vi "GetParam.vi"(8 "error in (no error)":errorcluster caption="entrée d'erreur (pas d'erreur)", 11 "Homogeneity_C_V_M.lvclass":refnum<class "Homogeneity_C_V_M.lvclass">) -> (0 "error out":errorcluster caption="sortie d'erreur", 2 "homogeneity_completeness_v_measure":cluster{"beta":dbl, "Returns":string}={"beta"=1.0, "Returns"="homogeneity"}, 3 "Homogeneity_C_V_M.lvclass":refnum<class "Homogeneity_C_V_M.lvclass">)   [LabVIEW 2020, in "Homogeneity_C_V_M.lvclass"]
doc: "Get parameters"
uses:
  Homogeneity_C_V_M.lvclass
  Homogeneity_C_V_M.lvclass/Homogeneity_C_V_M.ctl
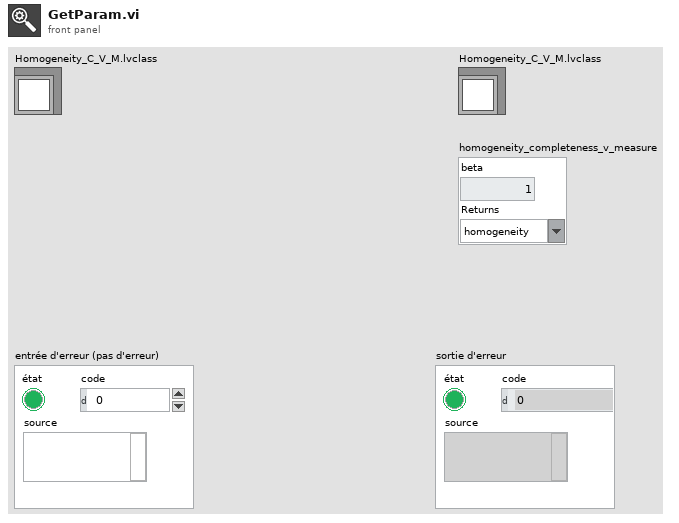
[diagram p1: front panel]
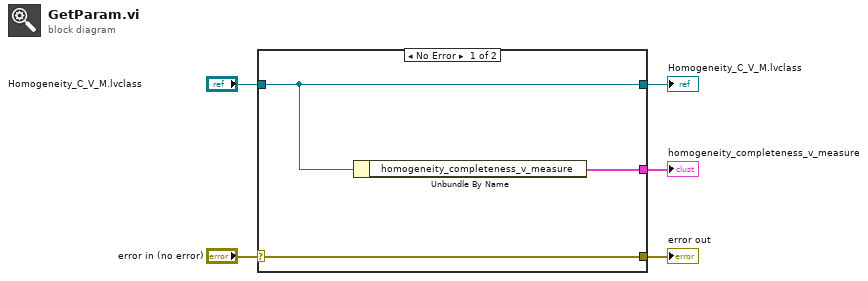
[diagram p0: block diagram]
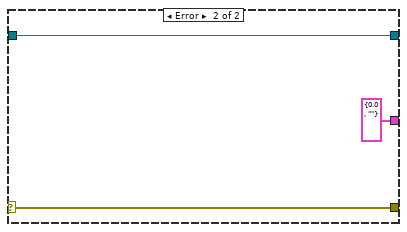
[diagram p2: hidden frame]
diagram:
  n1 = case shown="No Error" "error in (no error)" {
    selector: "error in (no error)" -> [w8 w10]
    tunnel: [w8 w10] -> w4
    tunnel: [w7 w11] -> w2
    tunnel: "Homogeneity_C_V_M.lvclass" -> [w7 w11]
    tunnel: [w6 cluster{"beta":dbl, "Returns":string} {"beta"=0.0, "Returns"=""} ("homogeneity_completeness_v_measure")] -> w1
    frame No Error {
      n2 = Unbundle By Name(w7) -> ("homogeneity_completeness_v_measure"=w6:cluster{"beta":dbl, "Returns":string})
    }
    frame Error {
    }
  }
  "error out" <- w4
  "Homogeneity_C_V_M.lvclass" <- w2
  "homogeneity_completeness_v_measure" <- w1
